vi "gaussmeter_setup.vi"(8 "error in (no error)":errorcluster, 10 "On/Off":bool, 11 "VISA Gaussmeter":refnum<visa-resource-name>) -> (0 "error out":errorcluster, 1 "Probe Sensitivity":dbl, 2 "Probe Type":u16, 3 "VISA Gaussmeter out":refnum<visa-resource-name>, 4 "Probe Field \nCompensation On":bool, 5 "Probe Serial Number":string)   [LabVIEW 2016]
uses:
  <instrlib>/Lake Shore 425/Lake Shore 425.lvlib
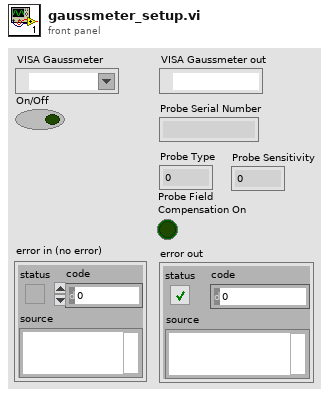
[diagram p1: front panel]
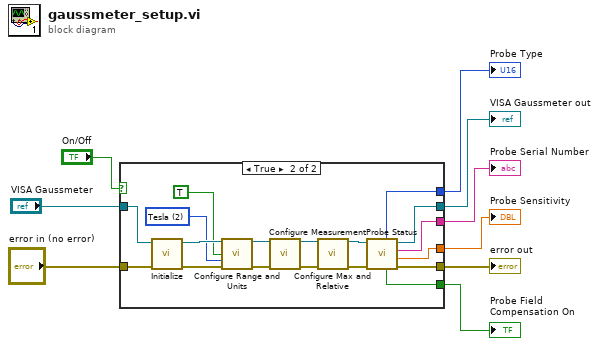
[diagram p0: block diagram]
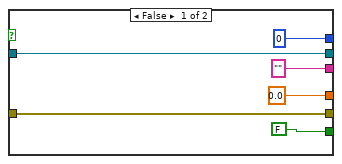
[diagram p2: hidden frame]
diagram:
  n1 = case shown="True" "On/Off" {
    tunnel: "VISA Gaussmeter" -> [w11 w33]
    tunnel: [w10 w30] -> w3
    tunnel: [FALSE w29] -> w4
    tunnel: [u16 0 ("Probe Type") w28] -> w6
    tunnel: ["" ("Probe Serial Number") w27] -> w1
    tunnel: [0.0 ("Probe Sensitivity") w26] -> w5
    tunnel: [w11 w19] -> w7
    tunnel: "error in (no error)" -> [w10 w16]
    frame False {
    }
    frame True {
      w17 = u16 2 items=["Gauss"=1, "Tesla"=2, "Oersted"=3, "Amp/meter"=4] ("Field Units (1:Gauss)")
      n2 = call <instrlib>:"Initialize.vi"("error in (no error)"=w16, "VISA resource name"=w33) -> ("error out"=w31:errorcluster, "VISA resource name out"=w32:refnum<visa-resource-name>)  [unwired: 8 in]
      n3 = call <instrlib>:"Configure Range and Units.vi"("VISA resource name"=w32, "Auto Range (F: Off)"=TRUE, "Field Units (1:Gauss)"=w17, "error in (no error)"=w31) -> ("VISA resource name out"=w25:refnum<visa-resource-name>, "error out"=w24:errorcluster)  [unwired: 10 in]
      n4 = call <instrlib>:"Configure Measurement.vi"("VISA resource name"=w25, "error in (no error)"=w24) -> ("VISA resource name out"=w21:refnum<visa-resource-name>, "error out"=w22:errorcluster)  [unwired: 12 in]
      n5 = call <instrlib>:"Configure Max and Relative.vi"("VISA resource name"=w21, "error in (no error)"=w22) -> ("VISA resource name out"=w20:refnum<visa-resource-name>, "error out"=w23:errorcluster)  [unwired: 12 in]
      n6 = call <instrlib>:"Probe Status.vi"("error in (no error)"=w23, "VISA resource name"=w20) -> ("error out"=w30:errorcluster, "Probe Sensitivity"=w26:dbl, "Probe Serial Number"=w27:string, "VISA resource name out"=w19:refnum<visa-resource-name>, "Probe Field \nCompensation On"=w29:bool, "Probe Type"=w28:u16)  [unwired: 4 in]
    }
  }
  "VISA Gaussmeter out" <- w7
  "Probe Type" <- w6
  "Probe Sensitivity" <- w5
  "Probe Field \nCompensation On" <- w4
  "error out" <- w3
  "Probe Serial Number" <- w1
